vi "HDLC Flag Check.vi"(2 "Min message Length":i32=158, 3 "Data in":bool[](array[boolean])) -> (0 "Detected":bool, 1 "Data Out":bool[](array[boolean]))   [LabVIEW 2019]
doc: "This VI detects flag and extract message between flags according to min message length.\nMin Message Length is require in order to make sure no consecutive flag should be detected.\nCurrently this is configured for detecting (01111110) 0x7E Pattern."
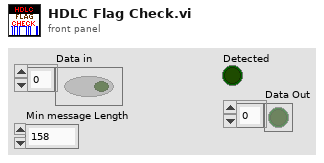
[diagram p1: front panel]
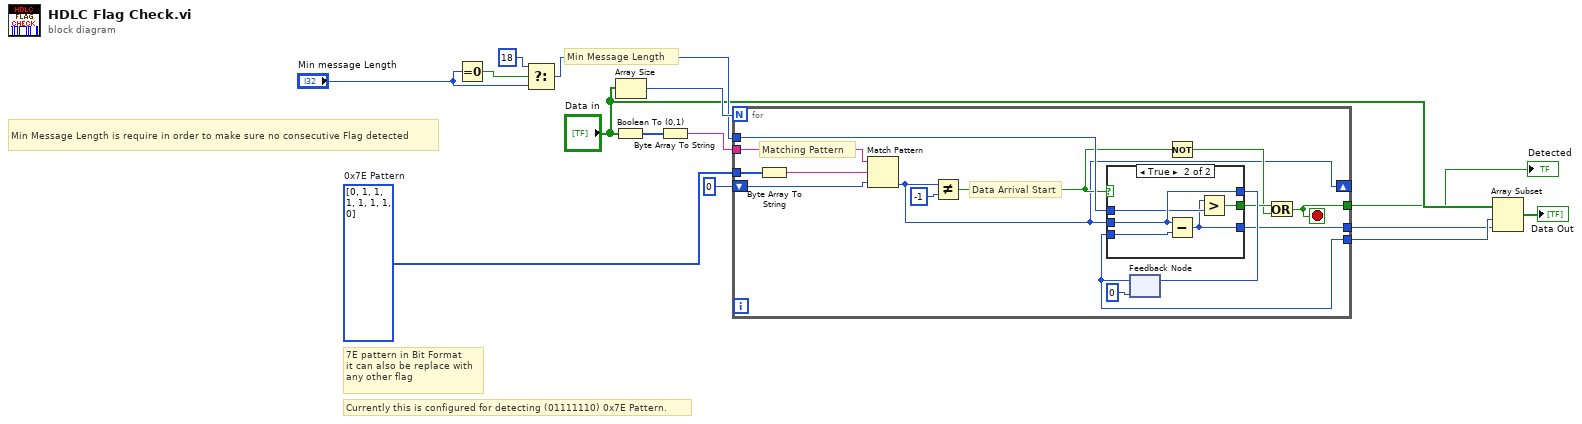
[diagram p0: block diagram]
diagram:
  w9 = i16[] [0, 1, 1, 1, 1, 1, 1, 0]  # 0x7E Pattern
  # "Currently this is configured for detecting (01111110) 0x7E Pattern."
  # "7E pattern in Bit Format\nit can also be replace with\nany other flag"
  # "Min Message Length is require in order to make sure no consecutive Flag detected"
  # "Min Message Length"
  n1 = Equal To 0?(x="Min message Length") -> (x = 0?=w14:bool)
  n2 = Select(t=18, s=w14, f="Min message Length") -> (s? t:f=w8:i32)
  n3 = Boolean To (0,1)(Boolean="Data in") -> (0, 1=w4:i16[])
  n4 = Array Size(array="Data in") -> (size(s)=w11:i32)
  n5 = Byte Array To String(unsigned byte array=w4) -> (string=w10:string)
  n6 = for {
    N: w11 -> [_]
    tunnel: w10 -> [w28]
    tunnel: w9 -> [w27]
    tunnel: w8 -> [w25]
    tunnel: [w19] -> w6
    tunnel: [w18] -> w5
    shift-right: [w17] -> _
    shift-left: 0 ("offset past match") -> [w16]
    tunnel: [w15] -> w1
    stop <- w15 stop-if-true
    # "Data Arrival Start"
    # "Matching Pattern"
    n7 = Byte Array To String(unsigned byte array=w27) -> (string=w29:string)
    n8 = Match Pattern(string=w28, regular expression=w29, offset (0)=w16) -> (offset past match=w17:i32)  [unwired: 3 out]
    n9 = Not Equal?(x=w17, y=-1) -> (x != y?=w21:bool)
    n10 = feedback #1(0) -> (w19:i32)
    n11 = case shown="True" w21 {
      tunnel: w17 -> [_ w33]
      tunnel: [w30 w33] -> w23
      tunnel: w19 -> [w30 w35]
      tunnel: [_ w34] -> w22
      tunnel: w25 -> [_ w32]
      tunnel: [_ w31] -> w18
      frame False {
      }
      frame True {
        n12 = Subtract(x=w33, y=w35) -> (x-y=w31:i32)
        n13 = Greater?(x=w31, y=w32) -> (0:w34:bool)
      }
    }
    n14 = feedback-in #1(w23) -> ()
    n15 = Not(x=w21) -> (.not. x?=w20:bool)
    n16 = Or(x=w22, y=w20) -> (x .or. y?=w15:bool)
  }
  "Detected" <- w1
  n17 = Array Subset(array="Data in", index=w6, length=w5) -> (→"Data Out":bool[])
